vi "Romi-Drive-System-Dash-Write.vi"(8 "error in (no error)":errorcluster) -> (0 "error out":errorcluster)   [LabVIEW 2019]
uses:
  Romi-Drive-System-Globals.vi
  <vilib>/Rock Robotics/Network Tables/NT Write Number.vi
  <vilib>/Rock Robotics/Network Tables/NT Write Numeric Array.vi
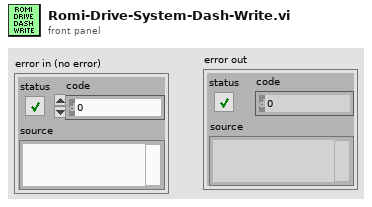
[diagram p1: front panel]
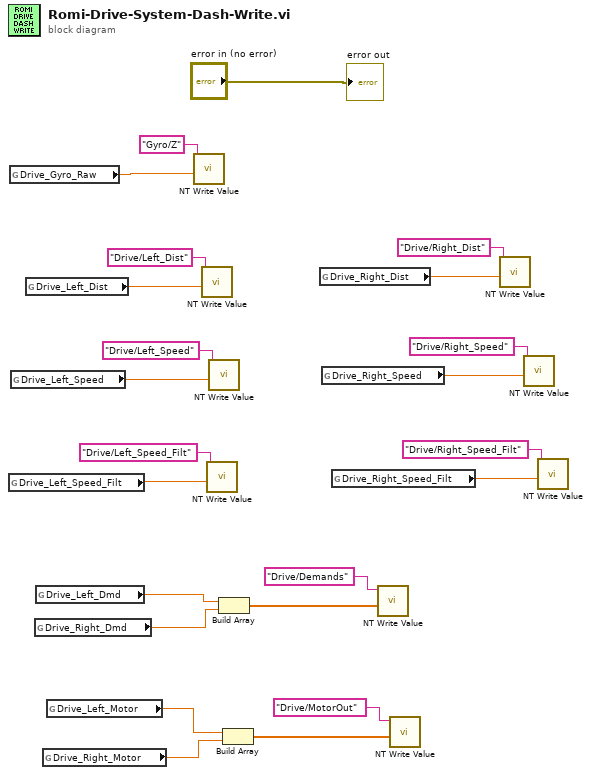
[diagram p0: block diagram]
diagram:
  n1 = global read "Romi-Drive-System-Globals.vi" "Drive_Left_Speed_Filt"() -> (w14:dbl)
  n2 = global read "Romi-Drive-System-Globals.vi" "Drive_Gyro_Raw"() -> (w15:dbl)
  n3 = global read "Romi-Drive-System-Globals.vi" "Drive_Left_Speed"() -> (w13:dbl)
  n4 = global read "Romi-Drive-System-Globals.vi" "Drive_Left_Dist"() -> (w11:dbl)
  n5 = global read "Romi-Drive-System-Globals.vi" "Drive_Right_Dmd"() -> (w5:dbl)
  n6 = global read "Romi-Drive-System-Globals.vi" "Drive_Left_Dmd"() -> (w6:dbl)
  n7 = global read "Romi-Drive-System-Globals.vi" "Drive_Right_Motor"() -> (w2:dbl)
  n8 = global read "Romi-Drive-System-Globals.vi" "Drive_Left_Motor"() -> (w3:dbl)
  n9 = call-poly <vilib>:"NT Write Value.vi"("Numeric"=w15, "Name"="Gyro/Z") -> ()  [unwired: 9 in, 1 out]
  n10 = call-poly <vilib>:"NT Write Value.vi"("Numeric"=w11, "Name"="Drive/Left_Dist") -> ()  [unwired: 9 in, 1 out]
  n11 = call-poly <vilib>:"NT Write Value.vi"("Numeric"=w14, "Name"="Drive/Left_Speed_Filt") -> ()  [unwired: 9 in, 1 out]
  n12 = call-poly <vilib>:"NT Write Value.vi"("Numeric"=w13, "Name"="Drive/Left_Speed") -> ()  [unwired: 9 in, 1 out]
  n13 = Build Array(w6, w5) -> (w7:dbl[])
  n14 = Build Array(w3, w2) -> (w1:dbl[])
  n15 = global read "Romi-Drive-System-Globals.vi" "Drive_Right_Dist"() -> (w10:dbl)
  n16 = global read "Romi-Drive-System-Globals.vi" "Drive_Right_Speed"() -> (w12:dbl)
  n17 = global read "Romi-Drive-System-Globals.vi" "Drive_Right_Speed_Filt"() -> (w9:dbl)
  n18 = call-poly <vilib>:"NT Write Value.vi"("Numeric Array"=w7, "Name"="Drive/Demands") -> ()  [unwired: 9 in, 1 out]
  n19 = call-poly <vilib>:"NT Write Value.vi"("Numeric Array"=w1, "Name"="Drive/MotorOut") -> ()  [unwired: 9 in, 1 out]
  n20 = call-poly <vilib>:"NT Write Value.vi"("Numeric"=w10, "Name"="Drive/Right_Dist") -> ()  [unwired: 9 in, 1 out]
  n21 = call-poly <vilib>:"NT Write Value.vi"("Numeric"=w12, "Name"="Drive/Right_Speed") -> ()  [unwired: 9 in, 1 out]
  n22 = call-poly <vilib>:"NT Write Value.vi"("Numeric"=w9, "Name"="Drive/Right_Speed_Filt") -> ()  [unwired: 9 in, 1 out]
  "error out" <- "error in (no error)"
